vi "Write Pages.vi"(5 "Pages":refnum<class "Page.lvclass">[](array[class]), 9 "PageSelector in":refnum<class "PageSelector.lvclass">) -> (3 "PageSelector out":refnum<class "PageSelector.lvclass">)   [LabVIEW 2014, in "Raspberry Pi Compatible Compiler for LabVIEW.lvlib" / "PageSelector.lvclass"]
uses:
  PageSelector.lvclass
  Page/Page.lvclass
  PageSelector.lvclass/PageSelector.ctl
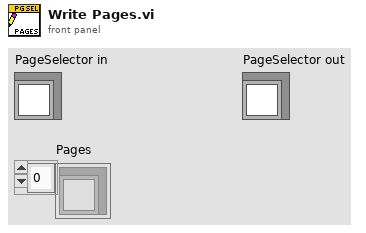
[diagram p1: front panel]
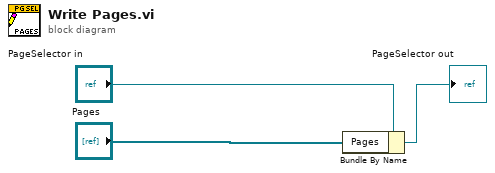
[diagram p0: block diagram]
diagram:
  n1 = Bundle By Name(cluster="PageSelector in", "Pages"="Pages") -> (→"PageSelector out":refnum<class "PageSelector.lvclass">)
